vi "A_times_x_fp.vi"(9 "Az_mat in":dbl[][](array[numeric]), 10 "x_k":dbl[](array[numeric])=[0.0, 0.0, 0.0, 0.0, 0.0, 0.0, 0.0, 0.0, 0.0, 0.0, 0.0, 0.0, 0.0, 0.0, 0.0, 0.0, 0.0, 0.0, 0.0, 0.0, 0.0, 0.0, 0.0, 0.0, 0.0, 0.0, 0.0, 0.0, 0.0, 0.0, 0.0, 0.0, 0.0, 0.0, 0.0, 0.0, 0.0, 0.0, 0.0, 0.0, 0.0, 0.0, 0.0, 0.0, 0.0, 0.0, 0.0, 0.0, 0.0, 0.0]) -> (2 "A*x":dbl[](array[numeric]), 3 "Az_vec out":dbl[](array[numeric]))   [LabVIEW 2017]
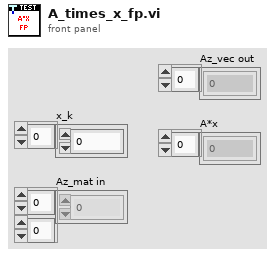
[diagram p1: front panel]
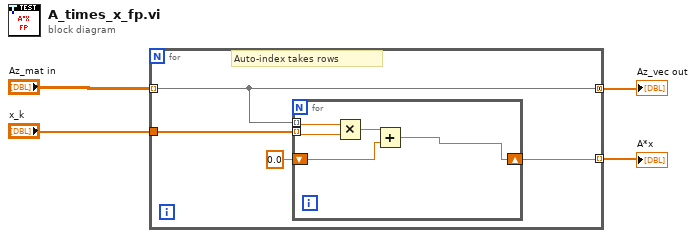
[diagram p0: block diagram]
diagram:
  n1 = for {
    tunnel: "Az_mat in" -> [w8] mode=indexing
    tunnel: [w8] -> w3 mode=concatenating
    tunnel: "x_k" -> [w7]
    tunnel: [w5] -> w4 mode=indexing
    # "Auto-index takes rows"
    n2 = for {
      tunnel: w8 -> [w13] mode=indexing
      tunnel: w7 -> [w12] mode=indexing
      shift-right: [w9] -> w5
      shift-left: 0.0 -> [w10]
      n3 = Multiply(x=w13, y=w12) -> (x*y=w11:dbl)
      n4 = Add(x=w11, y=w10) -> (x+y=w9:dbl)
    }
  }
  "A*x" <- w4
  "Az_vec out" <- w3
